vi "PH_PPMA_PowerUnit.check Waiting state.vi"(0 "i ref in":refnum<vi>, 5 "error in (no error)":errorcluster) -> (14 "i ref out":refnum<vi>, 17 "Waiting Time (s)":i32, 19 "error out":errorcluster)   [LabVIEW 2014, in "PH_PPMA_PowerUnit.lvlib"]
doc: "This VI calculates the state of the waiting time: if the waiting time is over, \"true\" is indicated. At the waiting time \"0\" appears at \"Waiting Time (s)\" in this case. Otherwise the remaining waiting is indicated in seconds. If an \"9999\" appears, an error occured by checking the waiting time.\n\n\"Required Device(s) off?\" is true if at least one device is even not switched on."
uses:
  PH_PPMA_PowerUnit.lvlib
  CSCore/BaseSM/BaseSM.lvlib
  lib.lib/DimLVEvent/LVDimInterface/LVDimInterface.lvlib
  PH_PowerUnit_BaseClass/PH_PowerUnit_BaseClass.lvlib
  PH_Common/PH_Common.lvlib
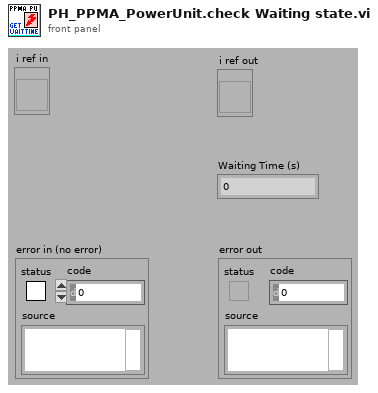
[diagram p1: front panel]
types:
  T1 = typedef "PH_PowerUnit_BaseClass.lvlib/PH_PowerUnit_BaseClass.i attribute.ctl" = cluster{"Constructor finished":bool, "PU":cluster{"In use":bool, "Service ID in use":i32, "GUI Ref":refnum<vi>}, "Enabling":cluster{"State":T2, "GUI Ref":refnum<vi>}, "Timing":cluster{"Last Shot":dbl, "Time between Shots [Sec]":dbl, "Waiting Time over?":bool, "Service ID Waiting Time":i32, "GUI Ref":refnum<vi>, "Instance":cluster{"Status":T3, "linked?":bool, "GUI Ref":refnum<vi>}}, "Sequencer":cluster{"SM State":string, "GUI Ref":refnum<vi>, "linked":bool}, "Subscribed Trendmssgs":cluster{"Tagname":string, "Status":T3, "linked?":bool, "Shot Condition":T3, "GUI Ref":refnum<vi>}[], "PP PU":T4, "Default Voltage (V)":dbl, "GUI Refs":T5, "PSDB data":cluster{"Shot Voltage [V]":dbl, "State TO SM":T6, "Write 2 early":bool}, "State TO SM":T6}
  T2 = typedef "PH_SystemInformation.lvlib/PH_SystemInformationEnabling State.ctl" = i32
  T3 = typedef "PH_StatusHandler.lvlib/PH_StatusHandler.Status.ctl" = i16
  T4 = typedef "PH_PP_Common.lvlib/PH_PP_Common.PUs.ctl" = enum16{"no Info", "PA-19mm-1", "PA-19mm-2", "PA-45mm-PILC", "PA-45mm-MAIN", "MA-PU-1", "MA-PU-2", "MA-PU-3", "MA-PU-4", "MA-PU-5", "MA-PU-6", "MA-FR", "MA-PILC", "PA-45mm-DP"}
  T5 = typedef "PH_PowerUnit_BaseClass.lvlib/PH_PowerUnit_BaseClass.GUI Refs.ctl" = cluster{"Delete Inst":refnum<vi>, "State TO SM":refnum<vi>, "State SM":refnum<vi>, "Fire":refnum<vi>}
  T6 = typedef "PH_PowerUnit_BaseClass.lvlib/PH_PowerUnit_BaseClass.SM States.ctl" = enum16{".", "Stand by", "Switch PU on", "Configure", "Set Default Voltage", "Set STANDBY", "Set READY", "Wait for Shot Cmd", "Open Dump Rods", "Open Ross Relais", "Close Ross Relais", "Switch PSU on", "Switch PSU off", "Charge", "Switch GD Channel on", "Close Dump Rods", "Rods-TO", "RR-TO", "PSU-TO", "Trigger-TO"}
  T7 = typedef "PH_PPMA_PowerUnit.lvlib/PH_PPMA_PowerUnit.i attribute.ctl" = cluster{"GUI Refs":cluster{"Rods":refnum<vi>, "Ignitron":refnum<vi>, "Rossrelais":refnum<vi>, "Set Voltage":refnum<vi>, "PSU":refnum<vi>, "EOC":refnum<vi>, "Trigger":refnum<vi>}, "Rods":T8, "PSU":T9, "Ross Relais":T10, "Ignitron":T11, "Trigger":cluster{"State Device":T3, "linked?":bool}, "Timing Settings":cluster{"Prdc Fast?":bool, "Default Value Periodic Interval":i32, "Mercury on since":dbl, "Warm up Time Mercury [s]":dbl}, "Set Voltage [V]":dbl}
  T8 = typedef "PH_PPMA_PowerUnit.lvlib/PH_PPMA_PowerUnit.Rods Attributes.ctl" = cluster{"Instancename":string, "Device Status":T3, "linked?":bool}
  T9 = typedef "PH_PP_Common.lvlib/PH_PP_Common.PSU Attributes.ctl" = cluster{"lower limit [V]":dbl, "upper limit [V]":dbl, "Voltage set":bool, "State Device":T3, "linked?":bool}
  T10 = typedef "PH_PP_Common.lvlib/PH_PP_Common.Ross Relais Attributes.ctl" = cluster{"State Device":T3, "linked?":bool}
  T11 = typedef "PH_PP_Common.lvlib/PH_PP_Common.Ignitron Attributes.ctl" = cluster{"State Device":T3, "linked?":bool}
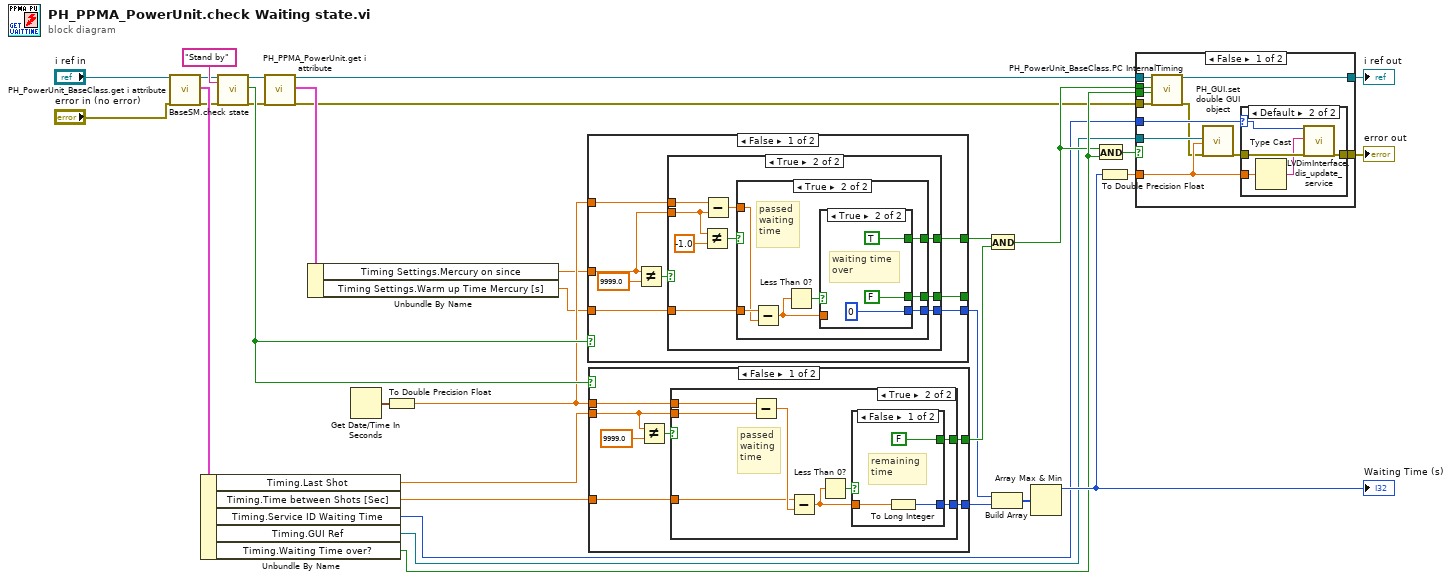
[diagram p0: block diagram]
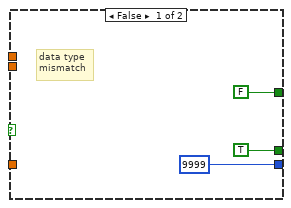
[diagram p4: hidden frame]
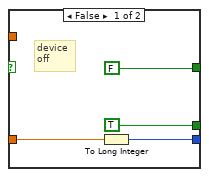
[diagram p5: hidden frame]
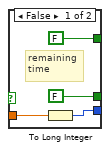
[diagram p6: hidden frame]
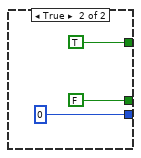
[diagram p7: hidden frame]
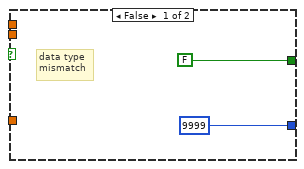
[diagram p8: hidden frame]
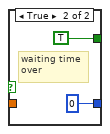
[diagram p9: hidden frame]
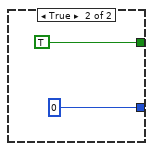
[diagram p10: hidden frame]
diagram:
  n1 = call "PH_PowerUnit_BaseClass.get i attribute.vi"("i ref in"="i ref in", "error in (no error)"="error in (no error)") -> ("i ref out"=w3:refnum<vi>, "i attribute"=w8:T1, "error out"=w2:errorcluster)  [unwired: 15 in]
  n2 = Unbundle By Name(w8) -> ("Timing.Last Shot"=w20:dbl, "Timing.Time between Shots [Sec]"=w29:dbl, "Timing.Service ID Waiting Time"=w9:i32, "Timing.GUI Ref"=w10:refnum<vi>, "Timing.Waiting Time over?"=w14:bool)
  n3 = call "BaseSM.check state.vi"("i ref in"=w3, "requestedState"="Stand by" ("requested state"), "error in (no error)"=w2) -> ("i ref out"=w7:refnum<vi>, "OK"=w26:bool, "error out"=w6:errorcluster)  [unwired: 11 in, 3 out]
  n4 = call "PH_PPMA_PowerUnit.get i attribute.vi"("i ref in"=w7, "error in (no error)"=w6) -> ("i ref out"=w5:refnum<vi>, "i attribute"=w19:T7, "error out"=w4:errorcluster)  [unwired: 15 in]
  n5 = Unbundle By Name(w19) -> ("Timing Settings.Mercury on since"=w18:dbl, "Timing Settings.Warm up Time Mercury [s]"=w1:dbl)
  n6 = Get Date/Time In Seconds() -> (seconds since 1Jan1904=w30:timestamp)
  n7 = To Double Precision Float(number=w30) -> (double precision float=w21:dbl)
  n8 = case shown="False" w26 {
    tunnel: [w37 FALSE] -> _
    tunnel: [w38 TRUE] -> w25
    tunnel: w1 -> [w39 _]
    tunnel: w18 -> [w34 _]
    tunnel: w21 -> [w40 _]
    tunnel: [w36 0] -> w23
    frame False {
      n9 = Not Equal?(x=w34, y=9999.0) -> (x != y?=w35:bool)
      n10 = case shown="True" w35 {
        tunnel: w34 -> [_ w45]
        tunnel: w40 -> [_ w47]
        tunnel: w39 -> [_ w44]
        tunnel: [FALSE w52] -> w38
        tunnel: [TRUE w51] -> w37
        tunnel: [9999 w50] -> w36
        frame False {
          # "data type\nmismatch"
        }
        frame True {
          n11 = Not Equal?(x=w45, y=-1.0) -> (x != y?=w48:bool)
          n12 = Subtract(x=w47, y=w45) -> (x-y=w46:dbl)
          n13 = case shown="True" w48 {
            tunnel: w46 -> [_ w57]
            tunnel: w44 -> [w54 w61]
            tunnel: [FALSE w60] -> w52
            tunnel: [TRUE w59] -> w51
            tunnel: [w53 w58] -> w50
            frame False {
              # "device \noff"
              n14 = To Long Integer(number=w54) -> (32bit integer=w53:i32)
            }
            frame True {
              # "passed\nwaiting\ntime"
              n15 = Subtract(x=w61, y=w57) -> (x-y=w63:dbl)
              n16 = Less Than 0?(x=w63) -> (x < 0?=w62:bool)
              n17 = case shown="True" w62 {
                tunnel: w63 -> [w67 _]
                tunnel: [w66 0] -> w58
                tunnel: [FALSE TRUE] -> w60
                tunnel: [FALSE FALSE] -> w59
                frame False {
                  # "remaining\ntime"
                  n18 = To Long Integer(number=w67) -> (32bit integer=w66:i32)
                }
                frame True {
                  # "waiting time\nover"
                }
              }
            }
          }
        }
      }
    }
    frame True {
    }
  }
  n19 = case "Check Waiting Time" shown="False" w26 {
    tunnel: [w78 TRUE] -> w28
    tunnel: w29 -> [w79 _]
    tunnel: w20 -> [w75 _]
    tunnel: w21 -> [w80 _]
    tunnel: [w77 0] -> w24
    frame False {
      n20 = Not Equal?(x=w75, y=9999.0) -> (x != y?=w76:bool)
      n21 = case shown="True" w76 {
        tunnel: w75 -> [_ w86]
        tunnel: w80 -> [_ w88]
        tunnel: w79 -> [_ w83]
        tunnel: [FALSE w90] -> w78
        tunnel: [9999 w89] -> w77
        frame False {
          # "data type\nmismatch"
        }
        frame True {
          # "passed\nwaiting\ntime"
          n22 = Subtract(x=w88, y=w86) -> (x-y=w87:dbl)
          n23 = Subtract(x=w83, y=w87) -> (x-y=w85:dbl)
          n24 = Less Than 0?(x=w85) -> (x < 0?=w84:bool)
          n25 = case shown="False" w84 {
            tunnel: w85 -> [w93 _]
            tunnel: [w92 0] -> w89
            tunnel: [FALSE TRUE] -> w90
            frame False {
              # "remaining\ntime"
              n26 = To Long Integer(number=w93) -> (32bit integer=w92:i32)
            }
            frame True {
              # "waiting time\nover"
            }
          }
        }
      }
    }
    frame True {
    }
  }
  n27 = And(x=w25, y=w28) -> (x .and. y?=w13:bool)
  n28 = Build Array(w23, w24) -> (w22:i32[])
  n29 = Array Max & Min(array=w22) -> (max value=w17:i32)  [unwired: 3 out]
  "Waiting Time (s)" <- w17
  n30 = And(x=w13, y=w14) -> (x .and. y?=w15:bool)
  n31 = To Double Precision Float(number=w17) -> (double precision float=w16:dbl)
  n32 = case shown="False" w15 {
    tunnel: w4 -> [w100 w115]
    tunnel: [w105 w115] -> w11
    tunnel: w5 -> [w108 w116]
    tunnel: [w107 w116] -> w12
    tunnel: w13 -> [w106 _]
    tunnel: w16 -> [w103 _]
    tunnel: w9 -> [w104 _]
    tunnel: w10 -> [w102 _]
    tunnel: w14 -> [w101 _]
    frame False {
      n33 = call "PH_PowerUnit_BaseClass.PC InternalTiming.vi"("i ref in"=w108, "Waiting Time over? new"=w106, "Waiting Time over? old"=w101, "error in (no error)"=w100) -> ("i ref out"=w107:refnum<vi>, "error out"=w99:errorcluster)  [unwired: 14 in]
      n34 = call "PH_GUI.set double GUI object.vi"("GUI object Ref"=w102, "value"=w103, "error in (no error)"=w99) -> ("error out"=w98:errorcluster)  [unwired: 16 in]
      n35 = case shown="Default" w104 {
        selector: w104 -> [_ w112]
        tunnel: [w109 w113] -> w105
        tunnel: w98 -> [w109 w114]
        tunnel: w103 -> [_ w110]
        frame -1 {
        }
        frame Default {
          n36 = Type Cast(x=w110) -> (*(type *) &x=w111:string)  [unwired: 1 in]
          n37 = call "LVDimInterface.dis_update_service.vi"("my_serviceID"=w112, "data"=w111, "error in (no error)"=w114) -> ("error out"=w113:errorcluster)  [unwired: 14 in, 2 out]
        }
      }
    }
    frame True {
    }
  }
  "i ref out" <- w12
  "error out" <- w11
